vi "Joystick Main.vi"(1 "Command List":T3(array[cluster]), 2 "Boolean Input":u32[](array[numeric])) -> ()   [LabVIEW 2018]
uses:
  States.ctl
  Buttons.ctl
  Swerve Drive/Vision Mode.ctl
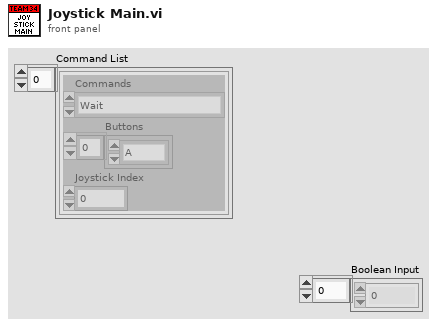
[diagram p1: front panel]
types:
  T1 = typedef "States.ctl" = enum16{"Wait", "Stop", "Limelight Follow", "NavX Reset", "Calibrate Wheels", "Pivot Forward", "Pivot Backward", "Flywheel Forward", "Flywheel Reverse", "FlyDrive Close", "FlyDrive Open", "Pivot Setpoint 0", "Pivot Setpoint 45", "Pivot Setpoint 90", "Low Goal", "Mid Goal", "High Goal", "Low Hatch", "Mid Hatch", "High Hatch"}
  T2 = typedef "Buttons.ctl" = enum16{"A", "B", "X", "Y", "LB", "RB", "Back", "Start", "LS", "RS"}
  T3 = cluster{"Commands":T1, "Buttons":T2[], "Joystick Index":dbl}[]
  T4 = typedef "Vision Mode.ctl" = enum16{"Track", "Keep Range", "Follow", "Stop"}
  T5 = enum16{"Low Hatch", "Low Goal", "Mid Hatch", "Mid Goal", "High Hatch", "High Goal"}
  T6 = enum16{"Open", "Raw Control", "Position Control"}
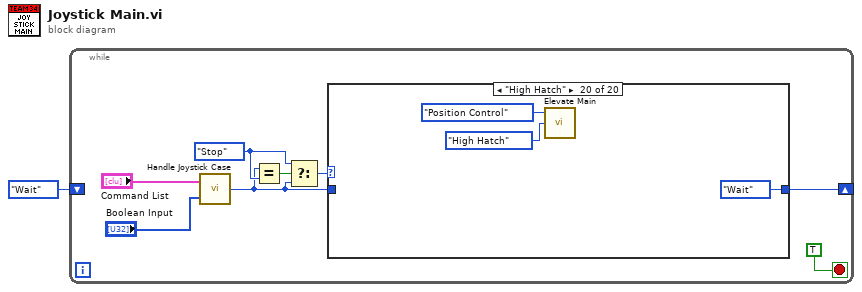
[diagram p0: block diagram]
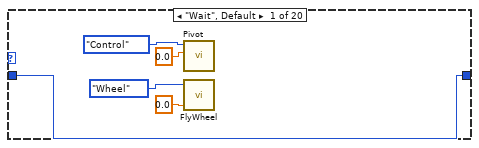
[diagram p2: hidden frame]
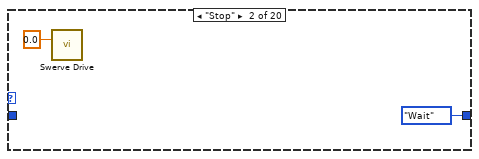
[diagram p3: hidden frame]
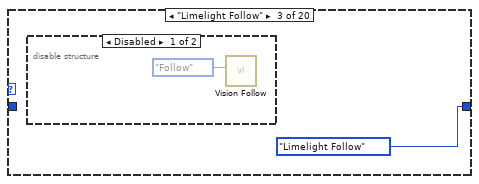
[diagram p4: hidden frame]
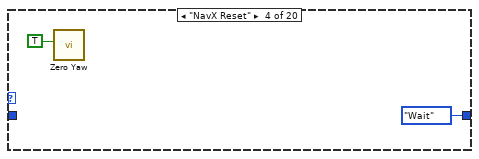
[diagram p6: hidden frame]
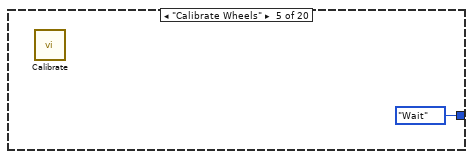
[diagram p7: hidden frame]
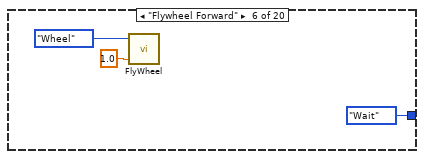
[diagram p8: hidden frame]
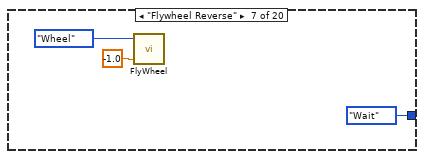
[diagram p9: hidden frame]
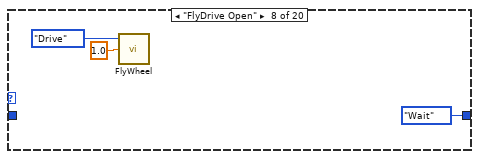
[diagram p10: hidden frame]
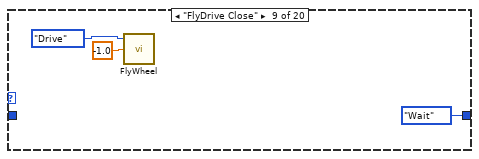
[diagram p11: hidden frame]
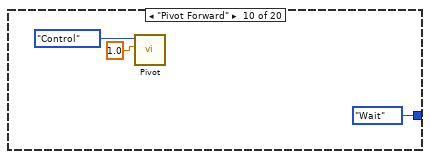
[diagram p12: hidden frame]
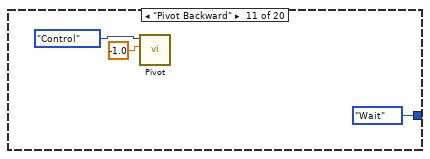
[diagram p13: hidden frame]
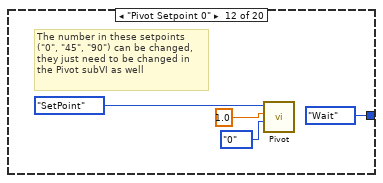
[diagram p14: hidden frame]
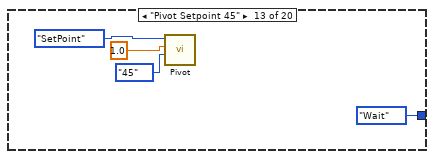
[diagram p15: hidden frame]
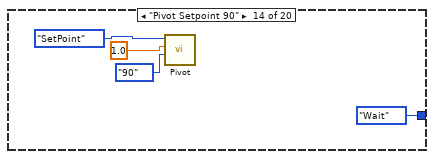
[diagram p16: hidden frame]
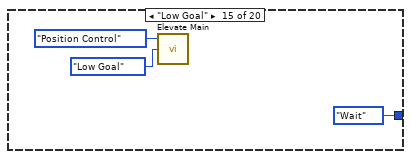
[diagram p17: hidden frame]
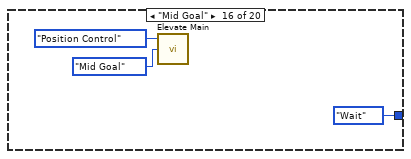
[diagram p18: hidden frame]
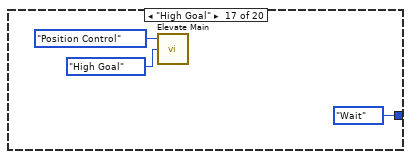
[diagram p19: hidden frame]
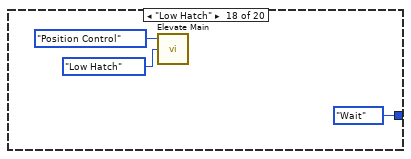
[diagram p20: hidden frame]
diagram:
  n1 = while {
    shift-right: [w4] -> _
    shift-left: States."Wait" ("Commands") -> [_]
    stop <- TRUE stop-if-true
    w6 = States."Stop" ("y")
    n2 = call "Handle Joystick Case.vi"("Boolean Input"="Boolean Input", "Command List"="Command List") -> ("Commands"=w3:T1)
    n3 = Equal?(x=w3, y=w6) -> (x = y?=w7:bool)
    n4 = Select(t=w6, s=w7, f=w3) -> (s? t:f=w5:T1)
    n5 = case shown="\"High Hatch\"" w5 {
      tunnel: [w14 States."Wait" ("f") States."Limelight Follow" ("f") States."Wait" ("Commands") States."Wait" ("Commands") States."Wait" ("Commands") States."Wait" ("Commands") States."Wait" ("Commands") States."Wait" ("Commands") States."Wait" ("Commands") States."Wait" ("Commands") States."Wait" ("Commands") States."Wait" ("Commands") States."Wait" ("Commands") States."Wait" ("Commands") States."Wait" ("Commands") States."Wait" ("Commands") States."Wait" ("Commands") States."Wait" ("Commands") States."Wait" ("Commands")] -> w4
      tunnel: w3 -> [w14 _ _ _ _ _ _ _ _ _ _ _ _ _ _ _ _ _ _ _]
      frame "Wait", Default {
        n6 = call "Pivot.vi"("Output"=0.0, "Enum"=enum16{"SetPoint", "Open", "Control"}."Control") -> ()  [unwired: 9 in, 1 out]
        n7 = call "FlyWheel.vi"("flyWheel Intake"=0.0, "Enum"=enum16{"Drive", "Wheel", "Open"}."Wheel") -> ()  [unwired: 2 in]
      }
      frame "Stop" {
        n8 = call "Swerve Drive.vi"("Y"=0.0 ("X")) -> ()  [unwired: 10 in, 5 out]
      }
      frame "Limelight Follow" {
        n9 = disable-structure shown="Disabled" {
          frame Disabled {
            n10 = call "Vision Follow.vi"("t"=Vision_Mode."Follow") -> ()  [unwired: 11 in]
          }
          frame Enabled {
          }
        }
      }
      frame "NavX Reset" {
        n11 = call <vilib>:"Zero Yaw.vi"("Zero"=TRUE) -> ()  [unwired: 11 in]
      }
      frame "Calibrate Wheels" {
        n12 = call "Calibrate.vi"() -> ()  [unwired: 12 in]
      }
      frame "Flywheel Forward" {
        n13 = call "FlyWheel.vi"("flyWheel Intake"=1.0, "Enum"=enum16{"Drive", "Wheel", "Open"}."Wheel") -> ()  [unwired: 2 in]
      }
      frame "Flywheel Reverse" {
        n14 = call "FlyWheel.vi"("flyWheel Intake"=-1.0, "Enum"=enum16{"Drive", "Wheel", "Open"}."Wheel") -> ()  [unwired: 2 in]
      }
      frame "FlyDrive Open" {
        n15 = call "FlyWheel.vi"("flyDrive movement"=1.0, "Enum"=enum16{"Drive", "Wheel", "Open"}."Drive") -> ()  [unwired: 2 in]
      }
      frame "FlyDrive Close" {
        n16 = call "FlyWheel.vi"("flyDrive movement"=-1.0, "Enum"=enum16{"Drive", "Wheel", "Open"}."Drive") -> ()  [unwired: 2 in]
      }
      frame "Pivot Forward" {
        n17 = call "Pivot.vi"("Output"=1.0, "Enum"=enum16{"SetPoint", "Open", "Control"}."Control") -> ()  [unwired: 9 in, 1 out]
      }
      frame "Pivot Backward" {
        n18 = call "Pivot.vi"("Output"=-1.0, "Enum"=enum16{"SetPoint", "Open", "Control"}."Control") -> ()  [unwired: 9 in, 1 out]
      }
      frame "Pivot Setpoint 0" {
        # "The number in these setpoints\n(\"0\", \"45\", \"90\") can be changed,\nthey just need to be changed in \nthe Pivot subVI as well"
        n19 = call "Pivot.vi"("setpointValue"=enum16{"90", "45", "0"}."0", "Output"=1.0, "Enum"=enum16{"SetPoint", "Open", "Control"}."SetPoint") -> ()  [unwired: 8 in, 1 out]
      }
      frame "Pivot Setpoint 45" {
        n20 = call "Pivot.vi"("setpointValue"=enum16{"90", "45", "0"}."45", "Output"=1.0, "Enum"=enum16{"SetPoint", "Open", "Control"}."SetPoint") -> ()  [unwired: 8 in, 1 out]
      }
      frame "Pivot Setpoint 90" {
        n21 = call "Pivot.vi"("setpointValue"=enum16{"90", "45", "0"}."90", "Output"=1.0, "Enum"=enum16{"SetPoint", "Open", "Control"}."SetPoint") -> ()  [unwired: 8 in, 1 out]
      }
      frame "Low Goal" {
        n22 = call "Elevate Main.vi"("Level"=T5."Low Goal", "Control Mode"=T6."Position Control") -> ()  [unwired: 2 in]
      }
      frame "Mid Goal" {
        n23 = call "Elevate Main.vi"("Level"=T5."Mid Goal", "Control Mode"=T6."Position Control") -> ()  [unwired: 2 in]
      }
      frame "High Goal" {
        n24 = call "Elevate Main.vi"("Level"=T5."High Goal", "Control Mode"=T6."Position Control") -> ()  [unwired: 2 in]
      }
      frame "Low Hatch" {
        n25 = call "Elevate Main.vi"("Level"=T5."Low Hatch", "Control Mode"=T6."Position Control") -> ()  [unwired: 2 in]
      }
      frame "Mid Hatch" {
        n26 = call "Elevate Main.vi"("Level"=T5."Mid Hatch", "Control Mode"=T6."Position Control") -> ()  [unwired: 2 in]
      }
      frame "High Hatch" {
        n27 = call "Elevate Main.vi"("Level"=T5."High Hatch", "Control Mode"=T6."Position Control") -> ()  [unwired: 2 in]
      }
    }
  }
